vi "App - analyze RUS V6.vi"() -> ()   [LabVIEW 2018] (continued)
"G (Hz)"=0.07528691046799785, "phi(rad)"=4.101336800213682, "Q"=8864.463580242193, "Norm  Ampl"=0.03358596834868616, "bg (V)"=0.3133810829522965-0.2519443963194782i, "4corners"={"z (-pi/2)"=-0.3079443963194782-0.3613810829522965i, "z(inf)"=0.3133810829522965-0.2519443963194782i, "z (pi/2)"=0.2039443963194782+0.3693810829522965i, "z center"=-0.05199999999999999+0.0040000000000000036i, "z(0)"=-0.4173810829522965+0.2599443963194782i, "radius"=0.4461063435849518}}, "timestamp(min)"=707.6166666671634, "timestamp"=timestamp(3493770278 s since 1904-01-01), "Magn Field(T)"=0.0}, {"temperature"=88.804, "lorentzian"={"A (VHz)"=0.0005765141419571238, "f (Hz)"=667.3663738953067, "G (Hz)"=0.07834180054863352, "phi(rad)"=4.144583024867645, "Q"=8518.649931731079, "Norm  Ampl"=0.034899318121872636, "bg (V)"=0.32357241448199386-0.2435691727610517i, "4corners"={"z (-pi/2)"=-0.29156917276105165-0.37957241448199386i, "z(inf)"=0.32357241448199386-0.2435691727610517i, "z (pi/2)"=0.1875691727610517+0.37157241448199385i, "z center"=-0.05199999999999999-0.0040000000000000036i, "z(0)"=-0.42757241448199385+0.2355691727610517i, "radius"=0.4454750577274212}}, "timestamp(min)"=708.9500000029802, "timestamp"=timestamp(3493770358 s since 1904-01-01), "Magn Field(T)"=0.0}, {"temperature"=88.687, "lorentzian"={"A (VHz)"=0.0005678584067974242, "f (Hz)"=667.3507898349178, "G (Hz)"=0.07706414952732094, "phi(rad)"=4.1398055492729045, "Q"=8659.678902942116, "Norm  Ampl"=0.033988854845615556, "bg (V)"=0.31870117348058796-0.2349611735919817i, "4corners"={"z (-pi/2)"=-0.2909611735919817-0.36670117348058795i, "z(inf)"=0.31870117348058796-0.2349611735919817i, "z (pi/2)"=0.18696117359198172+0.37470117348058796i, "z center"=-0.05199999999999999+0.0040000000000000036i, "z(0)"=-0.42270117348058794+0.24296117359198172i, "radius"=0.4410462589166154}}, "timestamp(min)"=710.2666666656733, "timestamp"=timestamp(3493770437 s since 1904-01-01), "Magn Field(T)"=0.0}, {"temperature"=88.566, "lorentzian"={"A (VHz)"=0.0005597284393444152, "f (Hz)"=667.3338926093543, "G (Hz)"=0.07546524086838977, "phi(rad)"=4.118302590104271, "Q"=8842.930664902726, "Norm  Ampl"=0.03370513681380475, "bg (V)"=0.3181055799932724-0.24600271249325478i, "4corners"={"z (-pi/2)"=-0.3020027124932548-0.36610557999327237i, "z(inf)"=0.3181055799932724-0.24600271249325478i, "z (pi/2)"=0.1980027124932548+0.3741055799932724i, "z center"=-0.05199999999999999+0.0040000000000000036i, "z(0)"=-0.42210557999327236+0.2540027124932548i, "radius"=0.4466312758821773}}, "timestamp(min)"=711.5833333358169, "timestamp"=timestamp(3493770516 s since 1904-01-01), "Magn Field(T)"=0.0}, {"temperature"=88.447, "lorentzian"={"A (VHz)"=0.0005697356914097864, "f (Hz)"=667.3173685004768, "G (Hz)"=0.07650786656191814, "phi(rad)"=4.128347855642436, "Q"=8722.205944148423, "Norm  Ampl"=0.03402552528878981, "bg (V)"=0.31901406796520765-0.24922529998140344i, "4corners"={"z (-pi/2)"=-0.29722529998140346-0.37501406796520764i, "z(inf)"=0.31901406796520765-0.24922529998140344i, "z (pi/2)"=0.19322529998140345+0.36701406796520764i, "z center"=-0.05199999999999999-0.0040000000000000036i, "z(0)"=-0.42301406796520763+0.24122529998140343i, "radius"=0.4447323761309278}}, "timestamp(min)"=712.9166666641831, "timestamp"=timestamp(3493770596 s since 1904-01-01), "Magn Field(T)"=0.0}, {"temperature"=88.332, "lorentzian"={"A (VHz)"=0.0005736346957575818, "f (Hz)"=667.3005746288229, "G (Hz)"=0.07673300638504786, "phi(rad)"=4.127101879531263, "Q"=8696.395541708536, "Norm  Ampl"=0.033990463573942475, "bg (V)"=0.3172396754700649-0.24871409423823745i, "4corners"={"z (-pi/2)"=-0.29671409423823747-0.37323967547006487i, "z(inf)"=0.3172396754700649-0.24871409423823745i, "z (pi/2)"=0.19271409423823746+0.36523967547006486i, "z center"=-0.05199999999999999-0.0040000000000000036i, "z(0)"=-0.42123967547006486+0.24071409423823745i, "radius"=0.44297056997060175}}, "timestamp(min)"=714.2333333343267, "timestamp"=timestamp(3493770675 s since 1904-01-01), "Magn Field(T)"=0.0}, {"temperature"=88.213, "lorentzian"={"A (VHz)"=0.000566647710639735, "f (Hz)"=667.2855690828252, "G (Hz)"=0.07598553132466843, "phi(rad)"=4.15143985044935, "Q"=8781.745122392707, "Norm  Ampl"=0.03357915756461218, "bg (V)"=0.32219190385022795-0.23909449154770343i, "4corners"={"z (-pi/2)"=-0.2870944915477034-0.37819190385022794i, "z(inf)"=0.32219190385022795-0.23909449154770343i, "z (pi/2)"=0.18309449154770344+0.37019190385022793i, "z center"=-0.05199999999999999-0.0040000000000000036i, "z(0)"=-0.4261919038502279+0.23109449154770342i, "radius"=0.4419151512034085}}, "timestamp(min)"=715.5666666701436, "timestamp"=timestamp(3493770755 s since 1904-01-01), "Magn Field(T)"=0.0}, {"temperature"=88.1, "lorentzian"={"A (VHz)"=0.0005776954308911229, "f (Hz)"=667.2692762902061, "G (Hz)"=0.07717942268646649, "phi(rad)"=4.16173072050711, "Q"=8645.68887747346, "Norm  Ampl"=0.033995543519673876, "bg (V)"=0.3233634137301181-0.23447736920675477i, "4corners"={"z (-pi/2)"=-0.28247736920675476-0.3793634137301181i, "z(inf)"=0.3233634137301181-0.23447736920675477i, "z (pi/2)"=0.17847736920675478+0.3713634137301181i, "z center"=-0.05199999999999999-0.0040000000000000036i, "z(0)"=-0.4273634137301181+0.22647736920675476i, "radius"=0.44047418776086594}}, "timestamp(min)"=716.8833333328366, "timestamp"=timestamp(3493770834 s since 1904-01-01), "Magn Field(T)"=0.0}, {"temperature"=87.983, "lorentzian"={"A (VHz)"=0.0005722338346167412, "f (Hz)"=667.2515590922309, "G (Hz)"=0.0764425608990404, "phi(rad)"=4.170141344014581, "Q"=8728.796513940535, "Norm  Ampl"=0.03354346259507517, "bg (V)"=0.32385977730037135-0.23045138061586795i, "4corners"={"z (-pi/2)"=-0.27845138061586794-0.37985977730037135i, "z(inf)"=0.32385977730037135-0.23045138061586795i, "z (pi/2)"=0.17445138061586796+0.37185977730037134i, "z center"=-0.05199999999999999-0.0040000000000000036i, "z(0)"=-0.42785977730037134+0.22245138061586794i, "radius"=0.43880610749523236}}, "timestamp(min)"=718.2000000029802, "timestamp"=timestamp(3493770913 s since 1904-01-01), "Magn Field(T)"=0.0}, {"temperature"=87.861, "lorentzian"={"A (VHz)"=0.0005955520518590209, "f (Hz)"=667.231376618077, "G (Hz)"=0.07844397285886262, "phi(rad)"=4.146322081912576, "Q"=8505.83355611741, "Norm  Ampl"=0.034365643115364705, "bg (V)"=0.3177566812895246-0.23895578116403757i, "4corners"={"z (-pi/2)"=-0.2869557811640375-0.3737566812895246i, "z(inf)"=0.3177566812895246-0.23895578116403757i, "z (pi/2)"=0.18295578116403757+0.3657566812895246i, "z center"=-0.05199999999999999-0.0040000000000000036i, "z(0)"=-0.4217566812895246+0.23095578116403756i, "radius"=0.43809156857972764}}, "timestamp(min)"=719.5333333313465, "timestamp"=timestamp(3493770993 s since 1904-01-01), "Magn Field(T)"=0.0}, {"temperature"=87.751, "lorentzian"={"A (VHz)"=0.000583124651348752, "f (Hz)"=667.2146515753702, "G (Hz)"=0.07660629595003704, "phi(rad)"=4.16535366394982, "Q"=8709.658172358711, "Norm  Ampl"=0.0335350855620341, "bg (V)"=0.32187688259715347-0.23170354643910587i, "4corners"={"z (-pi/2)"=-0.2797035464391059-0.37787688259715346i, "z(inf)"=0.32187688259715347-0.23170354643910587i, "z (pi/2)"=0.17570354643910588+0.36987688259715346i, "z center"=-0.05199999999999999-0.0040000000000000036i, "z(0)"=-0.42587688259715345+0.22370354643910587i, "radius"=0.43775887015743237}}, "timestamp(min)"=720.8500000014901, "timestamp"=timestamp(3493771072 s since 1904-01-01), "Magn Field(T)"=0.0}, {"temperature"=87.635, "lorentzian"={"A (VHz)"=0.0005990326023151825, "f (Hz)"=667.1959425135124, "G (Hz)"=0.07713621440132842, "phi(rad)"=4.17866165777404, "Q"=8649.581103918188, "Norm  Ampl"=0.03399022618486623, "bg (V)"=0.32736469704818216-0.2281798401488831i, "4corners"={"z (-pi/2)"=-0.2761798401488831-0.38336469704818216i, "z(inf)"=0.32736469704818216-0.2281798401488831i, "z (pi/2)"=0.1721798401488831+0.37536469704818215i, "z center"=-0.05199999999999999-0.0040000000000000036i, "z(0)"=-0.43136469704818214+0.2201798401488831i, "radius"=0.4406519875090067}}, "timestamp(min)"=722.1666666641831, "timestamp"=timestamp(3493771151 s since 1904-01-01), "Magn Field(T)"=0.0}, {"temperature"=87.523, "lorentzian"={"A (VHz)"=0.0006057654747408868, "f (Hz)"=667.1780248365252, "G (Hz)"=0.0772837615138755, "phi(rad)"=4.154776334690873, "Q"=8632.83582174944, "Norm  Ampl"=0.03403247684885089, "bg (V)"=0.3216524305694106-0.2370204010783713i, "4corners"={"z (-pi/2)"=-0.2850204010783713-0.3776524305694106i, "z(inf)"=0.3216524305694106-0.2370204010783713i, "z (pi/2)"=0.1810204010783713+0.3696524305694106i, "z center"=-0.05199999999999999-0.0040000000000000036i, "z(0)"=-0.4256524305694106+0.2290204010783713i, "radius"=0.44035740732858486}}, "timestamp(min)"=723.5, "timestamp"=timestamp(3493771231 s since 1904-01-01), "Magn Field(T)"=0.0}, {"temperature"=87.407, "lorentzian"={"A (VHz)"=0.0006112148090080954, "f (Hz)"=667.1610973636662, "G (Hz)"=0.07684505697732676, "phi(rad)"=4.185275210105214, "Q"=8681.89996346171, "Norm  Ampl"=0.03389817358475239, "bg (V)"=0.32924667269402136-0.22590328328648587i, "4corners"={"z (-pi/2)"=-0.27390328328648583-0.38524667269402135i, "z(inf)"=0.32924667269402136-0.22590328328648587i, "z (pi/2)"=0.16990328328648588+0.37724667269402135i, "z center"=-0.05199999999999999-0.0040000000000000036i, "z(0)"=-0.43324667269402134+0.21790328328648587i, "radius"=0.44112367038460387}}, "timestamp(min)"=724.8166666701436, "timestamp"=timestamp(3493771310 s since 1904-01-01), "Magn Field(T)"=0.0}, {"temperature"=87.293, "lorentzian"={"A (VHz)"=0.0006350154768766623, "f (Hz)"=667.1361303785343, "G (Hz)"=0.0770104032718294, "phi(rad)"=4.156400683489502, "Q"=8662.935162457128, "Norm  Ampl"=0.0341407512426947, "bg (V)"=0.32455231519635597-0.2379801797503247i, "4corners"={"z (-pi/2)"=-0.2859801797503247-0.38055231519635596i, "z(inf)"=0.32455231519635597-0.2379801797503247i, "z (pi/2)"=0.1819801797503247+0.37255231519635595i, "z center"=-0.05199999999999999-0.0040000000000000036i, "z(0)"=-0.42855231519635595+0.2299801797503247i, "radius"=0.44332648307509226}}, "timestamp(min)"=726.1499999985099, "timestamp"=timestamp(3493771390 s since 1904-01-01), "Magn Field(T)"=0.0}, {"temperature"=87.182, "lorentzian"={"A (VHz)"=0.0006171618328029761, "f (Hz)"=667.1181117945565, "G (Hz)"=0.07491261983076444, "phi(rad)"=4.154320976624089, "Q"=8905.283426232418, "Norm  Ampl"=0.03315493654368444, "bg (V)"=0.3234329017388911-0.23836826510269005i, "4corners"={"z (-pi/2)"=-0.28636826510269003-0.3794329017388911i, "z(inf)"=0.3234329017388911-0.23836826510269005i, "z (pi/2)"=0.18236826510269005+0.3714329017388911i, "z center"=-0.05199999999999999-0.0040000000000000036i, "z(0)"=-0.4274329017388911+0.23036826510269004i, "radius"=0.4425814584856992}}, "timestamp(min)"=727.4666666686535, "timestamp"=timestamp(3493771469 s since 1904-01-01), "Magn Field(T)"=0.0}, {"temperature"=87.068, "lorentzian"={"A (VHz)"=0.0006209755473867526, "f (Hz)"=667.0987327287644, "G (Hz)"=0.07577020215862286, "phi(rad)"=4.13814439529191, "Q"=8804.235883285772, "Norm  Ampl"=0.03316056448766872, "bg (V)"=0.3234492713577786-0.24172988900689188i, "4corners"={"z (-pi/2)"=-0.2817298890068919-0.3714492713577786i, "z(inf)"=0.3234492713577786-0.24172988900689188i, "z (pi/2)"=0.1937298890068919+0.3634492713577786i, "z center"=-0.043999999999999984-0.0040000000000000036i, "z(0)"=-0.4114492713577786+0.23372988900689187i, "radius"=0.437646509352687}}, "timestamp(min)"=728.7833333313465, "timestamp"=timestamp(3493771548 s since 1904-01-01), "Magn Field(T)"=0.0}, {"temperature"=86.958, "lorentzian"={"A (VHz)"=0.0006110556604820159, "f (Hz)"=667.0822028525415, "G (Hz)"=0.07532085232311952, "phi(rad)"=4.164222147727206, "Q"=8856.540815428114, "Norm  Ampl"=0.03300247944559944, "bg (V)"=0.3219601577129429-0.23233475863290984i, "4corners"={"z (-pi/2)"=-0.2803347586329098-0.3779601577129429i, "z(inf)"=0.3219601577129429-0.23233475863290984i, "z (pi/2)"=0.17633475863290984+0.3699601577129429i, "z center"=-0.05199999999999999-0.0040000000000000036i, "z(0)"=-0.4259601577129429+0.22433475863290983i, "radius"=0.4381586031982464}}, "timestamp(min)"=730.1166666671634, "timestamp"=timestamp(3493771628 s since 1904-01-01), "Magn Field(T)"=0.0}, {"temperature"=86.845, "lorentzian"={"A (VHz)"=0.0006113038691299176, "f (Hz)"=667.0647376572853, "G (Hz)"=0.07574099973177473, "phi(rad)"=4.1836995103504915, "Q"=8807.181579588254, "Norm  Ampl"=0.033183753683549984, "bg (V)"=0.3263041892781644-0.22498939176544208i, "4corners"={"z (-pi/2)"=-0.27298939176544207-0.3823041892781644i, "z(inf)"=0.3263041892781644-0.22498939176544208i, "z (pi/2)"=0.1689893917654421+0.3743041892781644i, "z center"=-0.05199999999999999-0.0040000000000000036i, "z(0)"=-0.4303041892781644+0.21698939176544207i, "radius"=0.4381214111388181}}, "timestamp(min)"=731.433333337307, "timestamp"=timestamp(3493771707 s since 1904-01-01), "Magn Field(T)"=0.0}, {"temperature"=86.732, "lorentzian"={"A (VHz)"=0.0006175376426682015, "f (Hz)"=667.0441866711889, "G (Hz)"=0.0741036591945461, "phi(rad)"=4.17351194093135, "Q"=9001.50132829449, "Norm  Ampl"=0.03278102830229572, "bg (V)"=0.32767735203270054-0.23101068010235828i, "4corners"={"z (-pi/2)"=-0.2790106801023583-0.38367735203270054i, "z(inf)"=0.32767735203270054-0.23101068010235828i, "z (pi/2)"=0.1750106801023583+0.37567735203270053i, "z center"=-0.05199999999999999-0.0040000000000000036i, "z(0)"=-0.4316773520327005+0.22301068010235828i, "radius"=0.44236720100737403}}, "timestamp(min)"=732.75, "timestamp"=timestamp(3493771786 s since 1904-01-01), "Magn Field(T)"=0.0}, {"temperature"=86.623, "lorentzian"={"A (VHz)"=0.0006285052671314143, "f (Hz)"=667.0271022203252, "G (Hz)"=0.07594321716369674, "phi(rad)"=4.212484466499658, "Q"=8783.234726315824, "Norm  Ampl"=0.033470084553526736, "bg (V)"=0.3347928660648436-0.21525795231311723i, "4corners"={"z (-pi/2)"=-0.2632579523131172-0.3907928660648436i, "z(inf)"=0.3347928660648436-0.21525795231311723i, "z (pi/2)"=0.15925795231311723+0.3827928660648436i, "z center"=-0.05199999999999999-0.0040000000000000036i, "z(0)"=-0.4387928660648436+0.20725795231311722i, "radius"=0.44072513390341983}}, "timestamp(min)"=734.0833333358169, "timestamp"=timestamp(3493771866 s since 1904-01-01), "Magn Field(T)"=0.0}, {"temperature"=86.512, "lorentzian"={"A (VHz)"=0.0006649470206808847, "f (Hz)"=667.0058178404381, "G (Hz)"=0.07805410313876843, "phi(rad)"=4.178881215672556, "Q"=8545.429273008267, "Norm  Ampl"=0.03459002019300002, "bg (V)"=0.3375685672355848-0.22936916717488998i, "4corners"={"z (-pi/2)"=-0.26936916717488996-0.3855685672355848i, "z(inf)"=0.3375685672355848-0.22936916717488998i, "z (pi/2)"=0.18136916717489+0.3775685672355848i, "z center"=-0.043999999999999984-0.0040000000000000036i, "z(0)"=-0.4255685672355848+0.22136916717488997i, "radius"=0.4431544121582459}}, "timestamp(min)"=735.3999999985099, "timestamp"=timestamp(3493771945 s since 1904-01-01), "Magn Field(T)"=0.0}, {"temperature"=86.405, "lorentzian"={"A (VHz)"=0.0006528045190258452, "f (Hz)"=666.9844113515632, "G (Hz)"=0.07653427367575434, "phi(rad)"=4.188368734592375, "Q"=8714.84603325974, "Norm  Ampl"=0.033665150998982166, "bg (V)"=0.3288460911604085-0.22409566572338693i, "4corners"={"z (-pi/2)"=-0.27209566572338695-0.3848460911604085i, "z(inf)"=0.3288460911604085-0.22409566572338693i, "z (pi/2)"=0.16809566572338694+0.3768460911604085i, "z center"=-0.05199999999999999-0.0040000000000000036i, "z(0)"=-0.4328460911604085+0.21609566572338693i, "radius"=0.439870261807255}}, "timestamp(min)"=736.7333333343267, "timestamp"=timestamp(3493772025 s since 1904-01-01), "Magn Field(T)"=0.0}, {"temperature"=86.294, "lorentzian"={"A (VHz)"=0.0006712967712834716, "f (Hz)"=666.9627164169844, "G (Hz)"=0.0758514496872024, "phi(rad)"=4.133754147443591, "Q"=8793.01211997157, "Norm  Ampl"=0.034020870334962316, "bg (V)"=0.3315051941986915-0.24928713946291586i, "4corners"={"z (-pi/2)"=-0.28928713946291584-0.3795051941986915i, "z(inf)"=0.3315051941986915-0.24928713946291586i, "z (pi/2)"=0.20128713946291588+0.3715051941986915i, "z center"=-0.043999999999999984-0.0040000000000000036i, "z(0)"=-0.4195051941986915+0.24128713946291586i, "radius"=0.44851971155802833}}, "timestamp(min)"=738.0500000044703, "timestamp"=timestamp(3493772104 s since 1904-01-01), "Magn Field(T)"=0.0}, {"temperature"=86.184, "lorentzian"={"A (VHz)"=0.0006656880154166683, "f (Hz)"=666.9433323926924, "G (Hz)"=0.07526321953860916, "phi(rad)"=4.119738991296172, "Q"=8861.477578042726, "Norm  Ampl"=0.033581794971741685, "bg (V)"=0.3260993716224481-0.253225090212679i, "4corners"={"z (-pi/2)"=-0.29322509021267906-0.3740993716224481i, "z(inf)"=0.3260993716224481-0.253225090212679i, "z (pi/2)"=0.20522509021267907+0.3660993716224481i, "z center"=-0.043999999999999984-0.0040000000000000036i, "z(0)"=-0.4140993716224481+0.24522509021267905i, "radius"=0.4461913159921974}}, "timestamp(min)"=739.3666666671634, "timestamp"=timestamp(3493772183 s since 1904-01-01), "Magn Field(T)"=0.0}, {"temperature"=86.077, "lorentzian"={"A (VHz)"=0.0006666643598218502, "f (Hz)"=666.9265821241922, "G (Hz)"=0.07601426481054148, "phi(rad)"=4.150143302494393, "Q"=8773.702985702026, "Norm  Ampl"=0.03382236181434309, "bg (V)"=0.33245238003541194-0.24119599197420452i, "4corners"={"z (-pi/2)"=-0.28119599197420453-0.38045238003541193i, "z(inf)"=0.33245238003541194-0.24119599197420452i, "z (pi/2)"=0.19319599197420453+0.3724523800354119i, "z center"=-0.043999999999999984-0.0040000000000000036i, "z(0)"=-0.4204523800354119+0.23319599197420451i, "radius"=0.4449475621272164}}, "timestamp(min)"=740.7000000029802, "timestamp"=timestamp(3493772263 s since 1904-01-01), "Magn Field(T)"=0.0}, {"temperature"=85.969, "lorentzian"={"A (VHz)"=0.0006725630187129924, "f (Hz)"=666.9065573278365, "G (Hz)"=0.07613991284832879, "phi(rad)"=4.139921437224611, "Q"=8758.96139592803, "Norm  Ampl"=0.03383447603734677, "bg (V)"=0.3295247101686151-0.24472001048915987i, "4corners"={"z (-pi/2)"=-0.28472001048915985-0.3775247101686151i, "z(inf)"=0.3295247101686151-0.24472001048915987i, "z (pi/2)"=0.19672001048915988+0.3695247101686151i, "z center"=-0.043999999999999984-0.0040000000000000036i, "z(0)"=-0.4175247101686151+0.23672001048915986i, "radius"=0.44437240300951314}}, "timestamp(min)"=742.0166666656733, "timestamp"=timestamp(3493772342 s since 1904-01-01), "Magn Field(T)"=0.0}, {"temperature"=85.861, "lorentzian"={"A (VHz)"=0.0006609657560129505, "f (Hz)"=666.8876756545675, "G (Hz)"=0.07451743556446012, "phi(rad)"=4.135619642082364, "Q"=8949.417953033111, "Norm  Ampl"=0.03305518137077315, "bg (V)"=0.32782980782843124-0.24589788836943288i, "4corners"={"z (-pi/2)"=-0.28589788836943286-0.37582980782843123i, "z(inf)"=0.32782980782843124-0.24589788836943288i, "z (pi/2)"=0.1978978883694329+0.3678298078284312i, "z center"=-0.043999999999999984-0.0040000000000000036i, "z(0)"=-0.4158298078284312+0.23789788836943287i, "radius"=0.44358989437014756}}, "timestamp(min)"=743.3333333358169, "timestamp"=timestamp(3493772421 s since 1904-01-01), "Magn Field(T)"=0.0}, {"temperature"=85.752, "lorentzian"={"A (VHz)"=0.000685177356303294, "f (Hz)"=666.8690344911956, "G (Hz)"=0.0768048531866786, "phi(rad)"=4.142116144215221, "Q"=8682.641875121253, "Norm  Ampl"=0.03421773382507842, "bg (V)"=0.3310141207484563-0.24451663667332432i, "4corners"={"z (-pi/2)"=-0.2845166366733243-0.3790141207484563i, "z(inf)"=0.3310141207484563-0.24451663667332432i, "z (pi/2)"=0.19651663667332434+0.3710141207484563i, "z center"=-0.043999999999999984-0.0040000000000000036i, "z(0)"=-0.4190141207484563+0.23651663667332432i, "radius"=0.4455152559423591}}, "timestamp(min)"=744.6666666641831, "timestamp"=timestamp(3493772501 s since 1904-01-01), "Magn Field(T)"=0.0}, {"temperature"=85.645, "lorentzian"={"A (VHz)"=0.0006570317642708686, "f (Hz)"=666.8501315259728, "G (Hz)"=0.07456835120073949, "phi(rad)"=4.108365651825874, "Q"=8942.803760415714, "Norm  Ampl"=0.03295267987103673, "bg (V)"=0.3197191912558564-0.24698790607990045i, "4corners"={"z (-pi/2)"=-0.29498790607990044-0.3597191912558564i, "z(inf)"=0.3197191912558564-0.24698790607990045i, "z (pi/2)"=0.20698790607990047+0.3677191912558564i, "z center"=-0.043999999999999984+0.0040000000000000036i, "z(0)"=-0.4077191912558564+0.25498790607990046i, "radius"=0.441912411102231}}, "timestamp(min)"=745.9833333343267, "timestamp"=timestamp(3493772580 s since 1904-01-01), "Magn Field(T)"=0.0}, {"temperature"=85.541, "lorentzian"={"A (VHz)"=0.0006674758378263185, "f (Hz)"=666.8344740108262, "G (Hz)"=0.07657160480826004, "phi(rad)"=4.159604046772095, "Q"=8708.639131707116, "Norm  Ampl"=0.03387404159939505, "bg (V)"=0.3324976658063025-0.23627781088496477i, "4corners"={"z (-pi/2)"=-0.2762778108849647-0.3804976658063025i, "z(inf)"=0.3324976658063025-0.23627781088496477i, "z (pi/2)"=0.18827781088496479+0.3724976658063025i, "z center"=-0.043999999999999984-0.0040000000000000036i, "z(0)"=-0.4204976658063025+0.22827781088496477i, "radius"=0.44238385344303166}}, "timestamp(min)"=747.3166666701436, "timestamp"=timestamp(3493772660 s since 1904-01-01), "Magn Field(T)"=0.0}, {"temperature"=85.433, "lorentzian"={"A (VHz)"=0.00067483946334777, "f (Hz)"=666.8133340701726, "G (Hz)"=0.0770265347392664, "phi(rad)"=4.149942916071108, "Q"=8656.930190710578, "Norm  Ampl"=0.033647342637348004, "bg (V)"=0.317536022353957-0.2369415784191966i, "4corners"={"z (-pi/2)"=-0.2849415784191966-0.373536022353957i, "z(inf)"=0.317536022353957-0.2369415784191966i, "z (pi/2)"=0.1809415784191966+0.365536022353957i, "z center"=-0.05199999999999999-0.0040000000000000036i, "z(0)"=-0.421536022353957+0.2289415784191966i, "radius"=0.43682794184164886}}, "timestamp(min)"=748.6333333328366, "timestamp"=timestamp(3493772739 s since 1904-01-01), "Magn Field(T)"=0.0}, {"temperature"=85.328, "lorentzian"={"A (VHz)"=0.0006839100759055985, "f (Hz)"=666.7935666574476, "G (Hz)"=0.07685381984981844, "phi(rad)"=4.15520036376655, "Q"=8676.127848432805, "Norm  Ampl"=0.033655710352043545, "bg (V)"=0.31968120300790964-0.23557224702626062i, "4corners"={"z (-pi/2)"=-0.2835722470262606-0.37568120300790964i, "z(inf)"=0.31968120300790964-0.23557224702626062i, "z (pi/2)"=0.17957224702626062+0.36768120300790963i, "z center"=-0.05199999999999999-0.0040000000000000036i, "z(0)"=-0.4236812030079096+0.2275722470262606i, "radius"=0.43791851098371987}}, "timestamp(min)"=749.9500000029802, "timestamp"=timestamp(3493772818 s since 1904-01-01), "Magn Field(T)"=0.0}, {"temperature"=85.224, "lorentzian"={"A (VHz)"=0.0006918096971641656, "f (Hz)"=666.7737931328093, "G (Hz)"=0.07743025734824358, "phi(rad)"=4.149525855521636, "Q"=8611.282152066027, "Norm  Ampl"=0.03371734359128283, "bg (V)"=0.31627716375248294-0.23636272328503305i, "4corners"={"z (-pi/2)"=-0.28436272328503304-0.37227716375248293i, "z(inf)"=0.31627716375248294-0.23636272328503305i, "z (pi/2)"=0.18036272328503306+0.3642771637524829i, "z center"=-0.05199999999999999-0.0040000000000000036i, "z(0)"=-0.4202771637524829+0.22836272328503304i, "radius"=0.43545436559300904}}, "timestamp(min)"=751.2833333313465, "timestamp"=timestamp(3493772898 s since 1904-01-01), "Magn Field(T)"=0.0}, {"temperature"=85.117, "lorentzian"={"A (VHz)"=0.0006987089466855211, "f (Hz)"=666.7536060450417, "G (Hz)"=0.07666284704999117, "phi(rad)"=4.144358590652548, "Q"=8697.219470733424, "Norm  Ampl"=0.03351893456612083, "bg (V)"=0.31656438446071555-0.23921530070664576i, "4corners"={"z (-pi/2)"=-0.28721530070664575-0.37256438446071555i, "z(inf)"=0.31656438446071555-0.23921530070664576i, "z (pi/2)"=0.18321530070664577+0.36456438446071554i, "z center"=-0.05199999999999999-0.0040000000000000036i, "z(0)"=-0.42056438446071553+0.23121530070664575i, "radius"=0.4372252773793207}}, "timestamp(min)"=752.6000000014901, "timestamp"=timestamp(3493772977 s since 1904-01-01), "Magn Field(T)"=0.0}, {"temperature"=85.014, "lorentzian"={"A (VHz)"=0.00073017153736958, "f (Hz)"=666.7360341780229, "G (Hz)"=0.0791126314816367, "phi(rad)"=4.177433959781578, "Q"=8427.681164072806, "Norm  Ampl"=0.03455920620628708, "bg (V)"=0.32380589709349605-0.2266997638651696i, "4corners"={"z (-pi/2)"=-0.2746997638651696-0.37980589709349605i, "z(inf)"=0.32380589709349605-0.2266997638651696i, "z (pi/2)"=0.1706997638651696+0.37180589709349604i, "z center"=-0.05199999999999999-0.0040000000000000036i, "z(0)"=-0.42780589709349603+0.2186997638651696i, "radius"=0.43683550349742595}}, "timestamp(min)"=753.9166666641831, "timestamp"=timestamp(3493773056 s since 1904-01-01), "Magn Field(T)"=0.0}, {"temperature"=84.907, "lorentzian"={"A (VHz)"=0.0007355828349611318, "f (Hz)"=666.714098457095, "G (Hz)"=0.07835939466609257, "phi(rad)"=4.154266083256125, "Q"=8508.413079224481, "Norm  Ampl"=0.03432647980443965, "bg (V)"=0.3195886391477811-0.2359967881677516i, "4corners"={"z (-pi/2)"=-0.2839967881677516-0.37558863914778107i, "z(inf)"=0.3195886391477811-0.2359967881677516i, "z (pi/2)"=0.1799967881677516+0.36758863914778106i, "z center"=-0.05199999999999999-0.0040000000000000036i, "z(0)"=-0.42358863914778105+0.2279967881677516i, "radius"=0.4380646373126373}}, "timestamp(min)"=755.25, "timestamp"=timestamp(3493773136 s since 1904-01-01), "Magn Field(T)"=0.0}, {"temperature"=84.805, "lorentzian"={"A (VHz)"=0.0007541138107820922, "f (Hz)"=666.6950355612224, "G (Hz)"=0.0793044480148079, "phi(rad)"=4.16249106282623, "Q"=8406.77984968429, "Norm  Ampl"=0.03504255712707177, "bg (V)"=0.3327318180890002-0.2349233311153916i, "4corners"={"z (-pi/2)"=-0.2749233311153916-0.3807318180890002i, "z(inf)"=0.3327318180890002-0.2349233311153916i, "z (pi/2)"=0.1869233311153916+0.3727318180890002i, "z center"=-0.043999999999999984-0.0040000000000000036i, "z(0)"=-0.4207318180890002+0.2269233311153916i, "radius"=0.44187379149941935}}, "timestamp(min)"=756.5666666701436, "timestamp"=timestamp(3493773215 s since 1904-01-01), "Magn Field(T)"=0.0}, {"temperature"=84.704, "lorentzian"={"A (VHz)"=0.0007311216213857258, "f (Hz)"=666.675358388109, "G (Hz)"=0.07753398797953004, "phi(rad)"=4.159703667226885, "Q"=8598.491780973782, "Norm  Ampl"=0.034101505233698926, "bg (V)"=0.3223442236464283-0.23489777524409902i, "4corners"={"z (-pi/2)"=-0.282897775244099-0.3783442236464283i, "z(inf)"=0.3223442236464283-0.23489777524409902i, "z (pi/2)"=0.17889777524409903+0.37034422364642827i, "z center"=-0.05199999999999999-0.0040000000000000036i, "z(0)"=-0.42634422364642827+0.22689777524409901i, "radius"=0.43982653443161157}}, "timestamp(min)"=757.8999999985099, "timestamp"=timestamp(3493773295 s since 1904-01-01), "Magn Field(T)"=0.0}, {"temperature"=84.597, "lorentzian"={"A (VHz)"=0.0007323955328732456, "f (Hz)"=666.6563167311539, "G (Hz)"=0.0768544938504149, "phi(rad)"=4.144181732136047, "Q"=8674.265919032592, "Norm  Ampl"=0.03387173640304755, "bg (V)"=0.3194730140460429-0.2411640353123799i, "4corners"={"z (-pi/2)"=-0.2891640353123799-0.3754730140460429i, "z(inf)"=0.3194730140460429-0.2411640353123799i, "z (pi/2)"=0.1851640353123799+0.3674730140460429i, "z center"=-0.05199999999999999-0.0040000000000000036i, "z(0)"=-0.4234730140460429+0.2331640353123799i, "radius"=0.4407255152701093}}, "timestamp(min)"=759.2166666686535, "timestamp"=timestamp(3493773374 s since 1904-01-01), "Magn Field(T)"=0.0}, {"temperature"=84.501, "lorentzian"={"A (VHz)"=0.0007333506518475584, "f (Hz)"=666.6383957613137, "G (Hz)"=0.07622384147794366, "phi(rad)"=4.130191799124422, "Q"=8745.798989338711, "Norm  Ampl"=0.03378638006202561, "bg (V)"=0.32622923299008494-0.24772682544579575i, "4corners"={"z (-pi/2)"=-0.28772682544579575-0.3742292329900849i, "z(inf)"=0.32622923299008494-0.24772682544579575i, "z (pi/2)"=0.19972682544579576+0.3662292329900849i, "z center"=-0.043999999999999984-0.0040000000000000036i, "z(0)"=-0.4142292329900849+0.23972682544579574i, "radius"=0.4432521296083212}}, "timestamp(min)"=760.5333333313465, "timestamp"=timestamp(3493773453 s since 1904-01-01), "Magn Field(T)"=0.0}, {"temperature"=84.397, "lorentzian"={"A (VHz)"=0.0007250782470453578, "f (Hz)"=666.6180927901069, "G (Hz)"=0.07362368121265518, "phi(rad)"=4.096676265251611, "Q"=9054.397740105418, "Norm  Ampl"=0.03269029871946489, "bg (V)"=0.3104800915070783-0.26043884193493727i, "4corners"={"z (-pi/2)"=-0.30843884193493726-0.3664800915070783i, "z(inf)"=0.3104800915070783-0.26043884193493727i, "z (pi/2)"=0.20443884193493728+0.35848009150707827i, "z center"=-0.05199999999999999-0.0040000000000000036i, "z(0)"=-0.41448009150707826+0.25243884193493726i, "radius"=0.4440188018450475}}, "timestamp(min)"=761.8666666671634, "timestamp"=timestamp(3493773533 s since 1904-01-01), "Magn Field(T)"=0.0}, {"temperature"=84.293, "lorentzian"={"A (VHz)"=0.0007593547216040537, "f (Hz)"=666.6002578587484, "G (Hz)"=0.07560760724100286, "phi(rad)"=4.085933881689177, "Q"=8816.576561323098, "Norm  Ampl"=0.03383046775040474, "bg (V)"=0.31848244372309686-0.2663282919673743i, "4corners"={"z (-pi/2)"=-0.30632829196737427-0.36648244372309685i, "z(inf)"=0.31848244372309686-0.2663282919673743i, "z (pi/2)"=0.2183282919673743+0.35848244372309684i, "z center"=-0.043999999999999984-0.0040000000000000036i, "z(0)"=-0.40648244372309683+0.2583282919673743i, "radius"=0.44744793526620286}}, "timestamp(min)"=763.183333337307, "timestamp"=timestamp(3493773612 s since 1904-01-01), "Magn Field(T)"=0.0}, {"temperature"=84.193, "lorentzian"={"A (VHz)"=0.0007488609817747594, "f (Hz)"=666.581167167379, "G (Hz)"=0.07473989204655404, "phi(rad)"=4.075929143471554, "Q"=8918.679822980992, "Norm  Ampl"=0.03365231566410544, "bg (V)"=0.31810056362730527-0.27161245964473i, "4corners"={"z (-pi/2)"=-0.31161245964473-0.36610056362730525i, "z(inf)"=0.31810056362730527-0.27161245964473i, "z (pi/2)"=0.22361245964473003+0.35810056362730525i, "z center"=-0.043999999999999984-0.0040000000000000036i, "z(0)"=-0.40610056362730523+0.26361245964473i, "radius"=0.4502590884549854}}, "timestamp(min)"=764.5, "timestamp"=timestamp(3493773691 s since 1904-01-01), "Magn Field(T)"=0.0}, {"temperature"=84.09, "lorentzian"={"A (VHz)"=0.0007704057058959121, "f (Hz)"=666.5603597826648, "G (Hz)"=0.075711318415688, "phi(rad)"=4.095160658837951, "Q"=8803.972427516836, "Norm  Ampl"=0.0341272478311757, "bg (V)"=0.3235842079326787-0.2648866243872285i, "4corners"={"z (-pi/2)"=-0.30488662438722847-0.3715842079326787i, "z(inf)"=0.3235842079326787-0.2648866243872285i, "z (pi/2)"=0.2168866243872285+0.3635842079326787i, "z center"=-0.043999999999999984-0.0040000000000000036i, "z(0)"=-0.4115842079326787+0.2568866243872285i, "radius"=0.45075490092250536}}, "timestamp(min)"=765.8333333358169, "timestamp"=timestamp(3493773771 s since 1904-01-01), "Magn Field(T)"=0.0}, {"temperature"=83.993, "lorentzian"={"A (VHz)"=0.0007765499522363316, "f (Hz)"=666.5413006512346, "G (Hz)"=0.0763481034904694, "phi(rad)"=4.10107868283753, "Q"=8730.292832151876, "Norm  Ampl"=0.03448377322577329, "bg (V)"=0.3258670481650503-0.2632290926405127i, "4corners"={"z (-pi/2)"=-0.3032290926405127-0.3738670481650503i, "z(inf)"=0.3258670481650503-0.2632290926405127i, "z (pi/2)"=0.2152290926405127+0.3658670481650503i, "z center"=-0.043999999999999984-0.0040000000000000036i, "z(0)"=-0.41386704816505027+0.2552290926405127i, "radius"=0.45166509250721504}}, "timestamp(min)"=767.1499999985099, "timestamp"=timestamp(3493773850 s since 1904-01-01), "Magn Field(T)"=0.0}, {"temperature"=83.89, "lorentzian"={"A (VHz)"=0.0007665748122083095, "f (Hz)"=666.5227729307114, "G (Hz)"=0.07546610066234899, "phi(rad)"=4.062113322899936, "Q"=8832.08178348677, "Norm  Ampl"=0.03406982041657331, "bg (V)"=0.3153235521042288-0.2773156702000033i, "4corners"={"z (-pi/2)"=-0.3173156702000033-0.3633235521042288i, "z(inf)"=0.3153235521042288-0.2773156702000033i, "z (pi/2)"=0.22931567020000332+0.3553235521042288i, "z center"=-0.043999999999999984-0.0040000000000000036i, "z(0)"=-0.40332355210422877+0.2693156702000033i, "radius"=0.4514586034994542}}, "timestamp(min)"=768.4833333343267, "timestamp"=timestamp(3493773930 s since 1904-01-01), "Magn Field(T)"=0.0}, {"temperature"=83.79, "lorentzian"={"A (VHz)"=0.0007670430927484451, "f (Hz)"=666.5025407776955, "G (Hz)"=0.07554097912991528, "phi(rad)"=4.048338646684716, "Q"=8823.059330902308, "Norm  Ampl"=0.034009766239806366, "bg (V)"=0.3105462857591947-0.2814733907319754i, "4corners"={"z (-pi/2)"=-0.3214733907319754-0.35854628575919467i, "z(inf)"=0.3105462857591947-0.2814733907319754i, "z (pi/2)"=0.23347339073197543+0.35054628575919466i, "z center"=-0.043999999999999984-0.0040000000000000036i, "z(0)"=-0.39854628575919465+0.2734733907319754i, "radius"=0.45021611622635194}}, "timestamp(min)"=769.8000000044703, "timestamp"=timestamp(3493774009 s since 1904-01-01), "Magn Field(T)"=0.0}, {"temperature"=83.692, "lorentzian"={"A (VHz)"=0.0007647830916334817, "f (Hz)"=666.4839616406631, "G (Hz)"=0.07558331971247774, "phi(rad)"=4.032528208883873, "Q"=8817.870982327811, "Norm  Ampl"=0.03412863564070823, "bg (V)"=0.30714207299413315-0.2798741816057033i, "4corners"={"z (-pi/2)"=-0.3278741816057033-0.34714207299413313i, "z(inf)"=0.30714207299413315-0.2798741816057033i, "z (pi/2)"=0.23987418160570334+0.35514207299413314i, "z center"=-0.043999999999999984+0.0040000000000000036i, "z(0)"=-0.3951420729941331+0.2878741816057033i, "radius"=0.4515366058349256}}, "timestamp(min)"=771.1166666671634, "timestamp"=timestamp(3493774088 s since 1904-01-01), "Magn Field(T)"=0.0}, {"temperature"=83.591, "lorentzian"={"A (VHz)"=0.0007660640978226073, "f (Hz)"=666.4635687138494, "G (Hz)"=0.07432529670564361, "phi(rad)"=4.005210008393842, "Q"=8966.847066259259, "Norm  Ampl"=0.03359054786770069, "bg (V)"=0.29956347396204774-0.2896214875438565i, "4corners"={"z (-pi/2)"=-0.3376214875438565-0.3395634739620477i, "z(inf)"=0.29956347396204774-0.2896214875438565i, "z (pi/2)"=0.24962148754385655+0.34756347396204773i, "z center"=-0.043999999999999984+0.0040000000000000036i, "z(0)"=-0.3875634739620477+0.29762148754385653i, "radius"=0.45193964042595086}}, "timestamp(min)"=772.4500000029802, "timestamp"=timestamp(3493774168 s since 1904-01-01), "Magn Field(T)"=0.0}, {"temperature"=83.495, "lorentzian"={"A (VHz)"=0.0007923326956308709, "f (Hz)"=666.4427909660764, "G (Hz)"=0.07645017941857793, "phi(rad)"=3.9568414021229756, "Q"=8717.347637828121, "Norm  Ampl"=0.036724329049090135, "bg (V)"=0.35365907482431364-0.3253832416764508i, "4corners"={"z (-pi/2)"=-0.3253832416764508-0.34565907482431363i, "z(inf)"=0.35365907482431364-0.3253832416764508i, "z (pi/2)"=0.3333832416764508+0.35365907482431364i, "z center"=0.0040000000000000036+0.0040000000000000036i, "z(0)"=-0.34565907482431363+0.3333832416764508i, "radius"=0.4803694291941174}}, "timestamp(min)"=773.7666666656733, "timestamp"=timestamp(3493774247 s since 1904-01-01), "Magn Field(T)"=0.0}, {"temperature"=83.396, "lorentzian"={"A (VHz)"=0.0007992909358441072, "f (Hz)"=666.4214629416866, "G (Hz)"=0.07562761312249623, "phi(rad)"=3.9207348865673355, "Q"=8811.880151000727, "Norm  Ampl"=0.03632129903000533, "bg (V)"=0.34146753303260685-0.337716516620038i, "4corners"={"z (-pi/2)"=-0.337716516620038-0.33346753303260684i, "z(inf)"=0.34146753303260685-0.337716516620038i, "z (pi/2)"=0.345716516620038+0.34146753303260685i, "z center"=0.0040000000000000036+0.0040000000000000036i, "z(0)"=-0.33346753303260684+0.345716516620038i, "radius"=0.4802650451386674}}, "timestamp(min)"=775.0833333358169, "timestamp"=timestamp(3493774326 s since 1904-01-01), "Magn Field(T)"=0.0}, {"temperature"=83.298, "lorentzian"={"A (VHz)"=0.000801456943825404, "f (Hz)"=666.4027073662497, "G (Hz)"=0.07619806299156674, "phi(rad)"=3.932828658603399, "Q"=8745.664669192498, "Norm  Ampl"=0.036623667084387954, "bg (V)"=0.35384048582971317-0.33387238466902386i, "4corners"={"z (-pi/2)"=-0.32587238466902385-0.33784048582971316i, "z(inf)"=0.35384048582971317-0.33387238466902386i, "z (pi/2)"=0.3498723846690239+0.34584048582971316i, "z center"=0.01200000000000001+0.0040000000000000036i, "z(0)"=-0.32984048582971315+0.34187238466902387i, "radius"=0.48063777012863557}}, "timestamp(min)"=776.4166666641831, "timestamp"=timestamp(3493774406 s since 1904-01-01), "Magn Field(T)"=0.0}, {"temperature"=83.202, "lorentzian"={"A (VHz)"=0.0008114289759602314, "f (Hz)"=666.3832582108636, "G (Hz)"=0.07809388258909512, "phi(rad)"=3.923610293808243, "Q"=8533.104465008582, "Norm  Ampl"=0.03772034393856336, "bg (V)"=0.35238507893272997-0.346694253244623i, "4corners"={"z (-pi/2)"=-0.330694253244623-0.34438507893272996i, "z(inf)"=0.35238507893272997-0.346694253244623i, "z (pi/2)"=0.354694253244623+0.33638507893272995i, "z center"=0.01200000000000001-0.0040000000000000036i, "z(0)"=-0.32838507893272995+0.338694253244623i, "radius"=0.4830127877882019}}, "timestamp(min)"=777.7333333343267, "timestamp"=timestamp(3493774485 s since 1904-01-01), "Magn Field(T)"=0.0}, {"temperature"=83.102, "lorentzian"={"A (VHz)"=0.0007831293066344564, "f (Hz)"=666.3597242998917, "G (Hz)"=0.07442620452206095, "phi(rad)"=3.8865417287402866, "Q"=8953.294455615744, "Norm  Ampl"=0.03547346853527881, "bg (V)"=0.33512118946399894-0.35437850516039704i, "4corners"={"z (-pi/2)"=-0.338378505160397-0.32712118946399893i, "z(inf)"=0.33512118946399894-0.35437850516039704i, "z (pi/2)"=0.36237850516039705+0.3191211894639989i, "z center"=0.01200000000000001-0.0040000000000000036i, "z(0)"=-0.3111211894639989+0.34637850516039703i, "radius"=0.4766260588334044}}, "timestamp(min)"=779.0500000044703, "timestamp"=timestamp(3493774564 s since 1904-01-01), "Magn Field(T)"=0.0}, {"temperature"=83.008, "lorentzian"={"A (VHz)"=0.0008282100382335496, "f (Hz)"=666.3423861780827, "G (Hz)"=0.08110599968317651, "phi(rad)"=3.8823519023008712, "Q"=8215.69783716382, "Norm  Ampl"=0.03846515133651509, "bg (V)"=0.3320521031725495-0.345981560851305i, "4corners"={"z (-pi/2)"=-0.337981560851305-0.3160521031725495i, "z(inf)"=0.3320521031725495-0.345981560851305i, "z (pi/2)"=0.361981560851305+0.3240521031725495i, "z center"=0.01200000000000001+0.0040000000000000036i, "z(0)"=-0.3080521031725495+0.353981560851305i, "radius"=0.4742577797791914}}, "timestamp(min)"=780.3833333328366, "timestamp"=timestamp(3493774644 s since 1904-01-01), "Magn Field(T)"=0.0}, {"temperature"=82.91, "lorentzian"={"A (VHz)"=0.0007451641386625461, "f (Hz)"=666.3219837699494, "G (Hz)"=0.07162019134956282, "phi(rad)"=3.858841846593944, "Q"=9303.54933733386, "Norm  Ampl"=0.03415064938942431, "bg (V)"=0.3254270265994654-0.3553469938487391i, "4corners"={"z (-pi/2)"=-0.34734699384873907-0.30942702659946536i, "z(inf)"=0.3254270265994654-0.3553469938487391i, "z (pi/2)"=0.3713469938487391+0.31742702659946537i, "z center"=0.01200000000000001+0.0040000000000000036i, "z(0)"=-0.30142702659946535+0.3633469938487391i, "radius"=0.47682990991663654}}, "timestamp(min)"=781.7000000029802, "timestamp"=timestamp(3493774723 s since 1904-01-01), "Magn Field(T)"=0.0}, {"temperature"=82.813, "lorentzian"={"A (VHz)"=0.0007370517746103769, "f (Hz)"=666.3027074087813, "G (Hz)"=0.07038271432673435, "phi(rad)"=3.8875074145442627, "Q"=9466.851538513218, "Norm  Ampl"=0.03359419640457404, "bg (V)"=0.3439218404495047-0.3545667940405476i, "4corners"={"z (-pi/2)"=-0.33056679404054756-0.3279218404495047i, "z(inf)"=0.3439218404495047-0.3545667940405476i, "z (pi/2)"=0.3705667940405476+0.31992184044950467i, "z center"=0.020000000000000018-0.0040000000000000036i, "z(0)"=-0.30392184044950465+0.3465667940405476i, "radius"=0.47730748559399533}}, "timestamp(min)"=783.0333333313465, "timestamp"=timestamp(3493774803 s since 1904-01-01), "Magn Field(T)"=0.0}, {"temperature"=82.719, "lorentzian"={"A (VHz)"=0.0007186859863431907, "f (Hz)"=666.2832044829721, "G (Hz)"=0.06930828334440148, "phi(rad)"=3.842055847945363, "Q"=9613.327185902557, "Norm  Ampl"=0.033076114874311065, "bg (V)"=0.3276101846222711-0.3608645481780698i, "4corners"={"z (-pi/2)"=-0.3448645481780698-0.3036101846222711i, "z(inf)"=0.3276101846222711-0.3608645481780698i, "z (pi/2)"=0.3848645481780698+0.3116101846222711i, "z center"=0.020000000000000018+0.0040000000000000036i, "z(0)"=-0.28761018462227106+0.3688645481780698i, "radius"=0.4772317719940016}}, "timestamp(min)"=784.3500000014901, "timestamp"=timestamp(3493774882 s since 1904-01-01), 
